vi "查詢接點名稱.vi"() -> ()   [LabVIEW 2015]
panel:
  out "error out":errorcluster
  out "Array":string[](array[string])
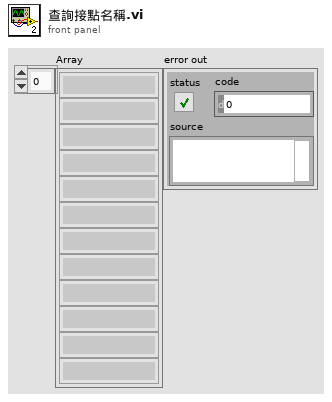
[diagram p1: front panel]
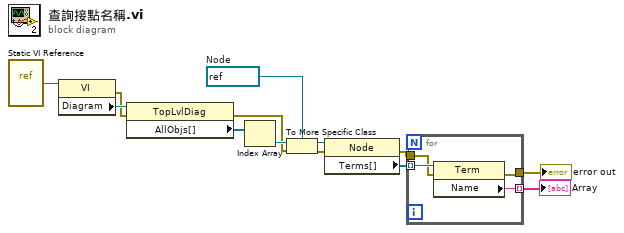
[diagram p0: block diagram]
diagram:
  w9 = refnum<vi> refnum  # Node
  n1 = vi-ref "Static VI Reference"() -> ("vi reference"=w1:refnum<vi>)
  n2 = property class="VI"(reference=w1) -> (error out=w6:errorcluster, "Diagram"=w13:refnum<vi>)  [unwired: 1 in, 1 out]
  n3 = property class="TopLvlDiag"(reference=w13, error in=w6) -> (error out=w5:errorcluster, "AllObjs[]"=w12:refnum<vi>[])  [unwired: 1 out]
  n4 = Index Array(array=w12) -> (element=w11:refnum<vi>)  [unwired: 1 in]
  n5 = To More Specific Class(target class=w9, reference=w11, error in=w5) -> (specific class reference=w10:refnum<vi>, error out=w4:errorcluster)
  n6 = property class="Node"(reference=w10, error in=w4) -> (error out=w3:errorcluster, "Terms[]"=w8:refnum<vi>[])  [unwired: 1 out]
  n7 = for {
    tunnel: w8 -> [w17] mode=indexing
    tunnel: [w16] -> w7 mode=indexing
    tunnel: w3 -> [w15]
    tunnel: [w14] -> w2
    n8 = property class="Term"(reference=w17, error in=w15) -> (error out=w14:errorcluster, "Name"=w16:string)  [unwired: 1 out]
  }
  "Array" <- w7
  "error out" <- w2
